vi "Check_matched_flow_meters.vi"   [LabVIEW 2016]
uses:
  <vilib>/Analysis/baseanly.llb/Mean (DBL).vi
  Globals/PressuresGlobal.vi
  <vilib>/Analysis/NI_AALBase.lvlib
panel:
  # "Checking to see if flow meters agree!"
types:
  T1 = enum16{"Release", "Create", "Send", "Wait", "Cancel"}
  T2 = cluster{"Flowboards":enum16{"A", "B", "C"}[], "Channels":enum16{"1", "2", "3", "4", "5", "6", "7", "8"}[], "States":bool[]}
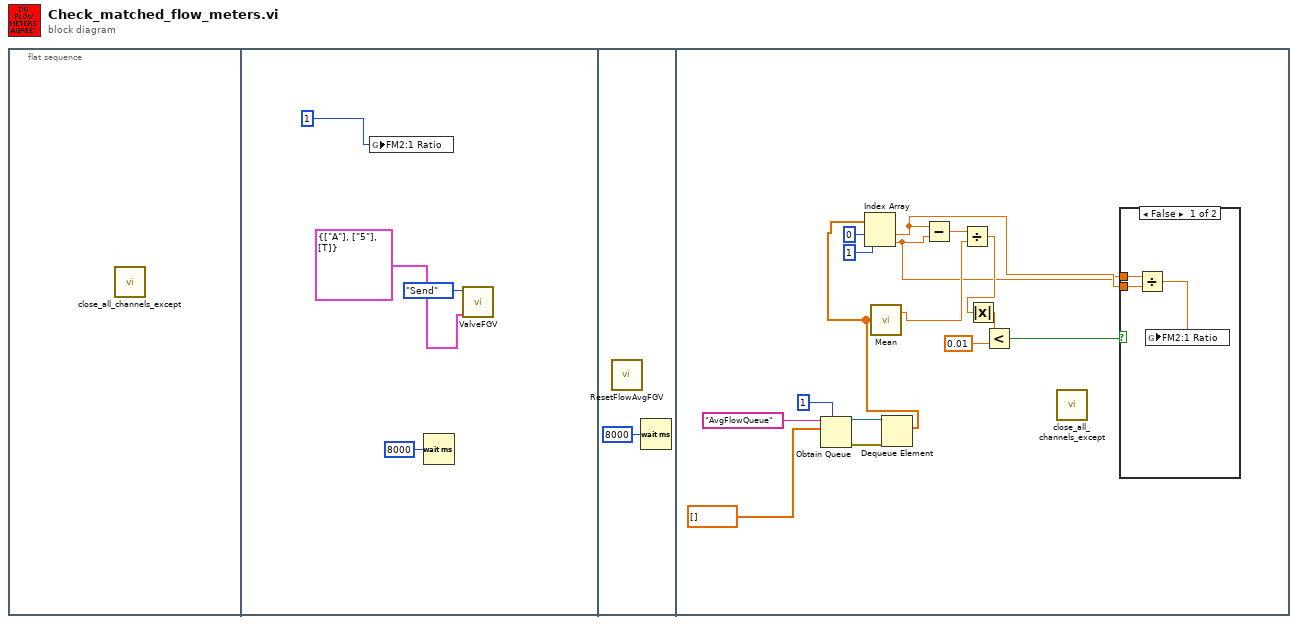
[diagram p0: block diagram]
diagram:
  n1 = flat-sequence {
    frame #0 {
      n2 = call "close_all_channels_except.vi"() -> ()  [unwired: 12 in]
    }
    frame #1 {
      n3 = global write "PressuresGlobal.vi" "FM2:1 Ratio"(1) -> ()
      n4 = Wait (ms)(milliseconds to wait=u32 8000) -> ()  [unwired: 1 out]
      n5 = call "ValveFGV.vi"("Valve Data"=T2 {"Flowboards"=[enum."A"], "Channels"=[enum."5"], "States"=[TRUE]}, "Action"=T1."Send") -> ()  [unwired: 6 in, 4 out]
    }
    frame #2 {
      n6 = call "ResetFlowAvgFGV.vi"() -> ()  [unwired: 11 in, 1 out]
      n7 = Wait (ms)(milliseconds to wait=u32 8000) -> ()  [unwired: 1 out]
    }
    frame #3 {
      n8 = Obtain Queue(max queue size (-1, unlimited)=1, name (unnamed)="AvgFlowQueue", element data type=dbl[] [] ("appended array")) -> (queue out=w8:refnum<queue>, error out=w7:errorcluster)  [unwired: 2 in, 1 out]
      n9 = Dequeue Element(queue=w8, error in (no error)=w7) -> (element=w6:dbl[])  [unwired: 1 in, 3 out]
      n10 = Index Array(array=w6, index #1=0 ("index"), index #2=1 ("index")) -> (element #1=w13:dbl, element #2=w12:dbl)
      n11 = call-poly <vilib>:"Mean.vi"("X"=w6) -> ("mean"=w18:dbl)  [unwired: 1 out]
      n12 = Subtract(x=w13, y=w12) -> (x-y=w19:dbl)
      n13 = Divide(x=w19, y=w18) -> (x/y=w17:dbl)
      n14 = Absolute Value(x=w17) -> (abs(x)=w16:dbl)
      n15 = Less?(x=w16, y=0.01) -> (x < y?=w14:bool)
      n16 = call "close_all_channels_except.vi"() -> ()  [unwired: 12 in]
      n17 = case shown="False" w14 {
        tunnel: w13 -> [w24 _]
        tunnel: w12 -> [w23 _]
        frame False {
          n18 = Divide(x=w23, y=w24) -> (x/y=w22:dbl)
          n19 = global write "PressuresGlobal.vi" "FM2:1 Ratio"(w22) -> ()
        }
        frame True {
        }
      }
    }
  }
